vi "Finish.vi"   [LabVIEW 2020]
doc: "This VIcloses device references, sends final commands to the network tables and the joysticks, and terminates all command and control loops."
uses:
  refnumbers.vi
  <vilib>/Rock Robotics/WPI/Utilities/WPI_GetSetVariantRefNum.vi
types:
  T1 = typedef "WPI_MotorControlDeviceRef.ctl" = cluster{"DeviceStatus":errorcluster, "Type":T2, "PWM":cluster{"PWM Channel":T3, "DeadBand":T4}, "CAN":cluster{"Device Number":u8, "SetOutput VI Ref":variant, "GetOutput VI Ref":variant, "Enable VI Ref":variant, "Disable VI Ref":variant, "Data":variant}, "Invert":bool, "DIO PWM":cluster{"PWM \"Enable\" Channel":T3, "DIOChannel":T5, "PWM Rate":dbl}}
  T2 = typedef "WPI_MotorControlType.ctl" = enum16{"PWM", "CAN", "DIO PWM"}
  T3 = typedef "FPGA_DIOPWMChannel.ctl" = enum8{"PWM 0", "PWM 1", "PWM 2", "PWM 3", "PWM 4", "PWM 5", "PWM 6", "PWM 7", "PWM 8", "PWM 9", "PWM MXP 0", "PWM MXP 1", "PWM MXP 2", "PWM MXP 3", "PWM MXP 4", "PWM MXP 5", "PWM MXP 6", "PWM MXP 7", "PWM MXP 8", "PWM MXP 9", "Invalid"}
  T4 = typedef "WPI_PWMDeadband.ctl" = cluster{"Name":string, "maxPositivePwm":i32, "minPositivePwm":i32, "centerPwm":i32, "maxNegativePwm":i32, "minNegativePwm":i32, "angularRange":u16}
  T5 = typedef "FPGA_DIOChannel.ctl" = enum8{"DIO 0", "DIO 1", "DIO 2", "DIO 3", "DIO 4", "DIO 5", "DIO 6", "DIO 7", "DIO 8", "DIO 9", "DIO MXP 0", "DIO MXP 1", "DIO MXP 2", "DIO MXP 3", "DIO MXP 4", "DIO MXP 5", "DIO MXP 6", "DIO MXP 7", "DIO MXP 8", "DIO MXP 9", "DIO MXP 10", "DIO MXP 11", "DIO MXP 12", "DIO MXP 13", "DIO MXP 14", "DIO MXP 15", "SPI Port CS1", "SPI Port CS2", "SPI Port CS3", "SPI Port MISO", "SPI Port MOSI", "Invalid"}
  T6 = typedef "WPI_SolenoidDevRef.ctl" = cluster{"DevStatus":errorcluster, "Pneumatics Control Module":u8, "Forward Solenoid Channel":T7, "Reverse Solenoid Channel":T7}
  T7 = typedef "WPI_SolenoidChannel.ctl" = enum8{"Solenoid 0", "Solenoid 1", "Solenoid 2", "Solenoid 3", "Solenoid 4", "Solenoid 5", "Solenoid 6", "Solenoid 7", "Solenoid 8", "Solenoid 9", "Solenoid 10", "Solenoid 11", "Solenoid 12", "Solenoid 13", "Solenoid 14", "Solenoid 15", "Invalid"}
  T8 = typedef "WPI_JoystickDevRef.ctl" = cluster{"Device":T9}
  T9 = typedef "WPI_JoystickDeviceEnum.ctl" = enum16{"USB 0", "USB 1", "USB 2", "USB 3", "USB 4", "USB 5"}
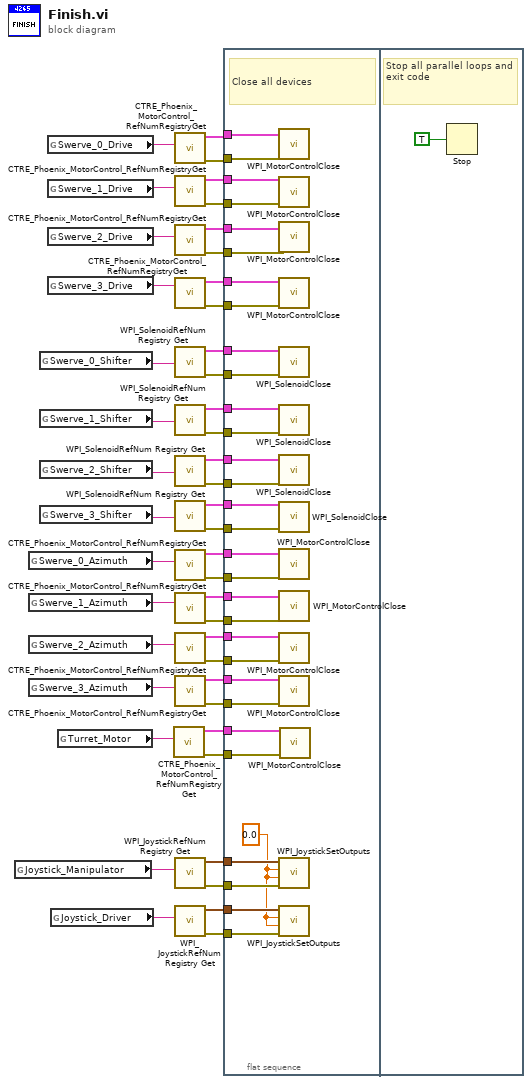
[diagram p0: block diagram]
diagram:
  n1 = global read "refnumbers.vi" "Joystick_Manipulator"() -> (w45:string)
  n2 = global read "refnumbers.vi" "Swerve_0_Azimuth"() -> (w24:string)
  n3 = global read "refnumbers.vi" "Swerve_1_Azimuth"() -> (w23:string)
  n4 = global read "refnumbers.vi" "Swerve_2_Azimuth"() -> (w22:string)
  n5 = global read "refnumbers.vi" "Swerve_3_Azimuth"() -> (w21:string)
  n6 = global read "refnumbers.vi" "Swerve_0_Shifter"() -> (w10:string)
  n7 = global read "refnumbers.vi" "Swerve_1_Shifter"() -> (w11:string)
  n8 = global read "refnumbers.vi" "Swerve_2_Shifter"() -> (w12:string)
  n9 = global read "refnumbers.vi" "Swerve_3_Shifter"() -> (w36:string)
  n10 = global read "refnumbers.vi" "Swerve_0_Drive"() -> (w33:string)
  n11 = global read "refnumbers.vi" "Swerve_1_Drive"() -> (w30:string)
  n12 = global read "refnumbers.vi" "Swerve_2_Drive"() -> (w28:string)
  n13 = global read "refnumbers.vi" "Swerve_3_Drive"() -> (w39:string)
  n14 = global read "refnumbers.vi" "Joystick_Driver"() -> (w40:string)
  n15 = global read "refnumbers.vi" "Turret_Motor"() -> (w3:string)
  n16 = call <vilib>:"CTRE_Phoenix_MotorControl_RefNumRegistryGet.vi"("refnum name"=w3) -> ("error out"=w1:errorcluster, "PhoenixMotorControlDevRef"=w2:T1)  [unwired: 9 in]
  n17 = call <vilib>:"CTRE_Phoenix_MotorControl_RefNumRegistryGet.vi"("refnum name"=w33) -> ("error out"=w31:errorcluster, "PhoenixMotorControlDevRef"=w32:T1)  [unwired: 9 in]
  n18 = call <vilib>:"CTRE_Phoenix_MotorControl_RefNumRegistryGet.vi"("refnum name"=w30) -> ("error out"=w25:errorcluster, "PhoenixMotorControlDevRef"=w29:T1)  [unwired: 9 in]
  n19 = call <vilib>:"CTRE_Phoenix_MotorControl_RefNumRegistryGet.vi"("refnum name"=w28) -> ("error out"=w26:errorcluster, "PhoenixMotorControlDevRef"=w27:T1)  [unwired: 9 in]
  n20 = call <vilib>:"CTRE_Phoenix_MotorControl_RefNumRegistryGet.vi"("refnum name"=w39) -> ("error out"=w37:errorcluster, "PhoenixMotorControlDevRef"=w38:T1)  [unwired: 9 in]
  n21 = call <vilib>:"WPI_SolenoidRefNum Registry Get.vi"("refnum name"=w10) -> ("error out"=w8:errorcluster, "SolenoidDevRef"=w9:T6)  [unwired: 9 in]
  n22 = call <vilib>:"WPI_SolenoidRefNum Registry Get.vi"("refnum name"=w11) -> ("error out"=w6:errorcluster, "SolenoidDevRef"=w7:T6)  [unwired: 9 in]
  n23 = call <vilib>:"WPI_SolenoidRefNum Registry Get.vi"("refnum name"=w12) -> ("error out"=w4:errorcluster, "SolenoidDevRef"=w5:T6)  [unwired: 9 in]
  n24 = call <vilib>:"WPI_SolenoidRefNum Registry Get.vi"("refnum name"=w36) -> ("error out"=w34:errorcluster, "SolenoidDevRef"=w35:T6)  [unwired: 9 in]
  n25 = call <vilib>:"CTRE_Phoenix_MotorControl_RefNumRegistryGet.vi"("refnum name"=w24) -> ("error out"=w16:errorcluster, "PhoenixMotorControlDevRef"=w20:T1)  [unwired: 9 in]
  n26 = call <vilib>:"CTRE_Phoenix_MotorControl_RefNumRegistryGet.vi"("refnum name"=w23) -> ("error out"=w15:errorcluster, "PhoenixMotorControlDevRef"=w19:T1)  [unwired: 9 in]
  n27 = call <vilib>:"CTRE_Phoenix_MotorControl_RefNumRegistryGet.vi"("refnum name"=w22) -> ("error out"=w14:errorcluster, "PhoenixMotorControlDevRef"=w18:T1)  [unwired: 9 in]
  n28 = call <vilib>:"CTRE_Phoenix_MotorControl_RefNumRegistryGet.vi"("refnum name"=w21) -> ("error out"=w13:errorcluster, "PhoenixMotorControlDevRef"=w17:T1)  [unwired: 9 in]
  n29 = call <vilib>:"WPI_JoystickRefNum Registry Get.vi"("refnum name"=w45) -> ("error out"=w43:errorcluster, "JoystickDevRef"=w44:T8)  [unwired: 9 in]
  n30 = call <vilib>:"WPI_JoystickRefNum Registry Get.vi"("refnum name"=w40) -> ("error out"=w41:errorcluster, "JoystickDevRef"=w42:T8)  [unwired: 9 in]
  n31 = flat-sequence {
    tunnel: w32 -> [w76]
    tunnel: w29 -> [w75]
    tunnel: w31 -> [w74]
    tunnel: w44 -> [w73]
    tunnel: w43 -> [w72]
    tunnel: w42 -> [w71]
    tunnel: w41 -> [w70]
    tunnel: w38 -> [w68]
    tunnel: w37 -> [w67]
    tunnel: w35 -> [w66]
    tunnel: w34 -> [w65]
    tunnel: w27 -> [w64]
    tunnel: w26 -> [w63]
    tunnel: w25 -> [w62]
    tunnel: w20 -> [w61]
    tunnel: w19 -> [w60]
    tunnel: w18 -> [w59]
    tunnel: w17 -> [w58]
    tunnel: w16 -> [w57]
    tunnel: w15 -> [w56]
    tunnel: w14 -> [w55]
    tunnel: w13 -> [w54]
    tunnel: w9 -> [w53]
    tunnel: w8 -> [w52]
    tunnel: w7 -> [w51]
    tunnel: w6 -> [w50]
    tunnel: w5 -> [w49]
    tunnel: w4 -> [w48]
    tunnel: w2 -> [w47]
    tunnel: w1 -> [w46]
    frame #0 {
      w69 = sgl 0.0 ("Left Rumble")
      # "Close all devices"
      n32 = call <vilib>:"WPI_MotorControlClose.vi"("error in"=w74, "MotorControlDevRef"=w76) -> ()  [unwired: 9 in, 1 out]
      n33 = call <vilib>:"WPI_MotorControlClose.vi"("error in"=w62, "MotorControlDevRef"=w75) -> ()  [unwired: 9 in, 1 out]
      n34 = call <vilib>:"WPI_MotorControlClose.vi"("error in"=w63, "MotorControlDevRef"=w64) -> ()  [unwired: 9 in, 1 out]
      n35 = call <vilib>:"WPI_MotorControlClose.vi"("error in"=w67, "MotorControlDevRef"=w68) -> ()  [unwired: 9 in, 1 out]
      n36 = call <vilib>:"WPI_SolenoidClose.vi"("error in (no error)"=w52, "SolenoidDevRef"=w53) -> ()  [unwired: 9 in, 1 out]
      n37 = call <vilib>:"WPI_SolenoidClose.vi"("error in (no error)"=w50, "SolenoidDevRef"=w51) -> ()  [unwired: 9 in, 1 out]
      n38 = call <vilib>:"WPI_SolenoidClose.vi"("error in (no error)"=w48, "SolenoidDevRef"=w49) -> ()  [unwired: 9 in, 1 out]
      n39 = call <vilib>:"WPI_SolenoidClose.vi"("error in (no error)"=w65, "SolenoidDevRef"=w66) -> ()  [unwired: 9 in, 1 out]
      n40 = call <vilib>:"WPI_MotorControlClose.vi"("error in"=w57, "MotorControlDevRef"=w61) -> ()  [unwired: 9 in, 1 out]
      n41 = call <vilib>:"WPI_MotorControlClose.vi"("error in"=w56, "MotorControlDevRef"=w60) -> ()  [unwired: 9 in, 1 out]
      n42 = call <vilib>:"WPI_MotorControlClose.vi"("error in"=w55, "MotorControlDevRef"=w59) -> ()  [unwired: 9 in, 1 out]
      n43 = call <vilib>:"WPI_MotorControlClose.vi"("error in"=w54, "MotorControlDevRef"=w58) -> ()  [unwired: 9 in, 1 out]
      n44 = call <vilib>:"WPI_JoystickSetOutputs.vi"("error in (no error)"=w72, "Right Rumble"=w69, "Left Rumble"=w69, "JoystickDevRef"=w73) -> ()  [unwired: 6 in, 2 out]
      n45 = call <vilib>:"WPI_JoystickSetOutputs.vi"("error in (no error)"=w70, "Right Rumble"=w69, "Left Rumble"=w69, "JoystickDevRef"=w71) -> ()  [unwired: 6 in, 2 out]
      n46 = call <vilib>:"WPI_MotorControlClose.vi"("error in"=w46, "MotorControlDevRef"=w47) -> ()  [unwired: 9 in, 1 out]
    }
    frame #1 {
      # "Stop all parallel loops and exit code"
      n47 = Stop(stop? (T)=TRUE ("Quit")) -> ()
    }
  }
